vi "TestServerComm1.vi"() -> ()   [LabVIEW 2017]
uses:
  <vilib>/addons/InsightCM/MessageBus/Base/controls/ConnectionInfo.ctl
  <vilib>/NI/Software Watchdog/Pound/Pound.lvclass
  <vilib>/addons/Qbus/Qbus.lvclass
  <vilib>/addons/TraceLogger/TraceLogger.lvlib
  <vilib>/addons/InsightCM/Devices/Shared/Common/ServerComm/ServerComm.lvlib
  <vilib>/addons/TimerProcess/TimerProcess.lvlib
panel:
  out "log":i32(listbox)=-1
  in  "stop":bool
  in  "connection info":T1={"ClientName"="Bop9068", "TransceiverHost"="10.2.64.56", "TransceiverPort"=6342, "Password"="password"}
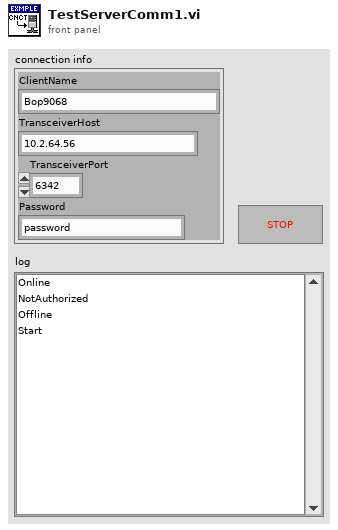
[diagram p1: front panel]
types:
  T1 = typedef "ConnectionInfo.ctl" = cluster{"ClientName":string, "TransceiverHost":string, "TransceiverPort":u16, "Password":string}
  T2 = typedef "ServerComm.lvlib/ConnectionStatus.ctl" = enum16{"Offline", "NotAuthorized", "Online"}
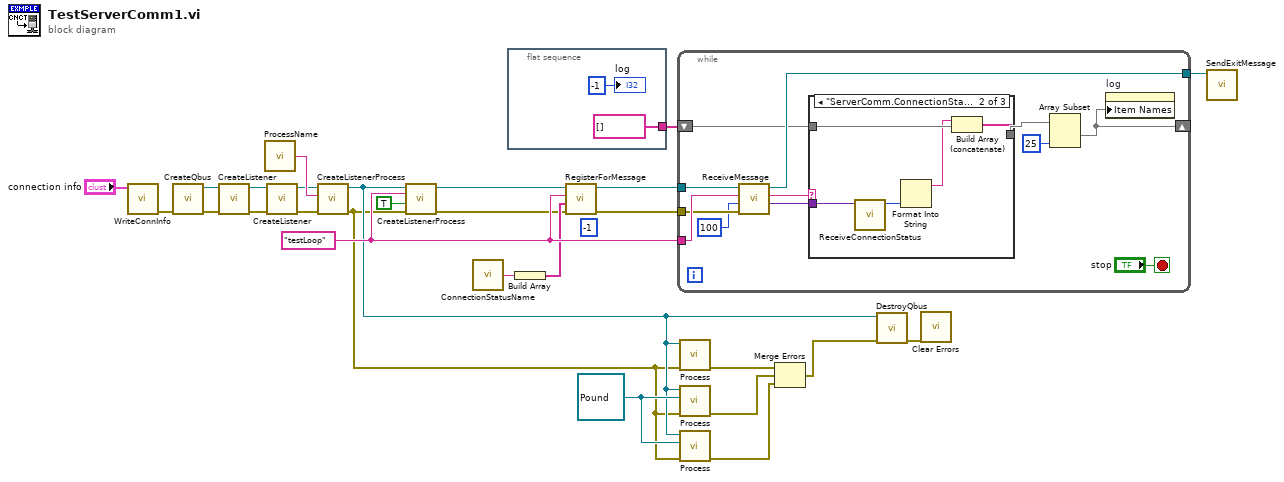
[diagram p0: block diagram]
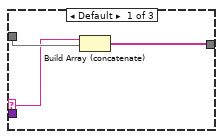
[diagram p2: hidden frame]
diagram:
  (unwired) -1 ("timeout (-1)")
  w14 = refnum<class "Pound.lvclass"> refnum ("Pound in")
  w17 = "testLoop" ("ProcessName")
  n1 = call <vilib>:"WriteConnInfo.vi"("connection info"="connection info") -> ("error out"=w22:errorcluster)  [unwired: 10 in]
  n2 = call <vilib>:"CreateQbus.vi"("error in (no error)"=w22) -> ("error out"=w11:errorcluster, "Qbus"=w12:refnum<class "Qbus.lvclass">)  [unwired: 9 in]
  n3 = call <vilib>:"CreateListener.vi"("error in (no error)"=w11, "Qbus in"=w12) -> ("error out"=w9:errorcluster, "Qbus out"=w10:refnum<class "Qbus.lvclass">)  [unwired: 8 in]
  n4 = call <vilib>:"ProcessName.vi"() -> ("process name"=w27:string)  [unwired: 5 in]
  n5 = call <vilib>:"CreateListener.vi"("error in (no error)"=w9, "qbus in"=w10) -> ("error out"=w7:errorcluster, "qbus out"=w8:refnum<class "Qbus.lvclass">)  [unwired: 8 in]
  n6 = call <vilib>:"CreateListenerProcess.vi"("error in (no error)"=w7, "process name"=w27, "Qbus in"=w8) -> ("error in (no error)"=w5:errorcluster, "Qbus out"=w6:refnum<class "Qbus.lvclass">)  [unwired: 7 in]
  n7 = call <vilib>:"CreateListenerProcess.vi"("error in (no error)"=w5, "master"=TRUE ("Master"), "process name"=w17, "Qbus in"=w6) -> ("error in (no error)"=w2:errorcluster, "Qbus out"=w1:refnum<class "Qbus.lvclass">)  [unwired: 6 in]
  n8 = call <vilib>:"ConnectionStatusName.vi"() -> ("message name"=w15:string)  [unwired: 5 in]
  n9 = flat-sequence {
    tunnel: [string[] []] -> w19
    frame #0 {
      "log" <- -1 ("Listbox")
    }
  }
  n10 = Build Array(w15) -> (w16:string[])
  n11 = call <vilib>:"RegisterForMessage.vi"("error in (no error)"=w2, "message names"=w16, "process name"=w17, "Qbus in"=w1) -> ("error in (no error)"=w3:errorcluster, "Qbus out"=w4:refnum<class "Qbus.lvclass">)  [unwired: 6 in]
  n12 = while {
    tunnel: w4 -> [w41]
    tunnel: w17 -> [w40]
    tunnel: w3 -> [w39]
    tunnel: [w35] -> w20
    shift-right: [w31] -> _
    shift-left: w19 -> [w34]
    stop <- "stop" stop-if-true
    n13 = call <vilib>:"ReceiveMessage.vi"("error in (no error)"=w39, "timeout (0)"=100, "process name"=w40, "Qbus in"=w41) -> ("message value"=w30:variant, "message name"=w36:string, "Qbus out"=w35:refnum<class "Qbus.lvclass">)  [unwired: 2 in, 3 out]
    n14 = case shown="\"ServerComm.ConnectionStatus\"" w36 {
      selector: w36 -> [w43 _ _]
      tunnel: [w42 w48 w50] -> w32
      tunnel: w34 -> [w44 w49 w50]
      tunnel: w30 -> [_ w46 _]
      frame Default {
        n15 = Build Array (concatenate)(w43, w44) -> (w42:string[])
      }
      frame "ServerComm.ConnectionStatus" {
        n16 = call <vilib>:"ReceiveConnectionStatus.vi"("body"=w46) -> ("status"=w45:T2)  [unwired: 7 in, 3 out]
        n17 = Format Into String(w45) -> (resulting string=w47:string)  [unwired: 3 in, 1 out]
        n18 = Build Array (concatenate)(w47, w49) -> (w48:string[])
      }
      frame "" {
      }
    }
    n19 = Array Subset(array=w32, length=25) -> (w31:string[])  [unwired: 1 in]
    n20 = property on="log" class="LstBox (strict)"("Item Names"=w31) -> ()  [unwired: 2 in, 2 out]
  }
  n21 = call <vilib>:"Process.vi"("error in (no error)"=w5, "qbus in"=w6) -> ("error out"=w25:errorcluster)  [unwired: 9 in]
  n22 = call <vilib>:"Process.vi"("error in (no error)"=w5, "Pound in"=w14, "Qbus in"=w6) -> ("error out"=w23:errorcluster)  [unwired: 8 in]
  n23 = call <vilib>:"Process.vi"("error in (no error)"=w5, "pound in"=w14, "qbus in"=w6) -> ("error out"=w13:errorcluster)  [unwired: 8 in]
  n24 = Merge Errors(w25, w23, w13) -> (w24:errorcluster)
  n25 = call <vilib>:"DestroyQbus.vi"("error in (no error)"=w24, "Qbus"=w6) -> ("error in (no error)"=w18:errorcluster)  [unwired: 9 in]
  n26 = call <vilib>:"Clear Errors.vi"("error in (no error)"=w18) -> ()  [unwired: 5 in, 2 out]
  n27 = call <vilib>:"SendExitMessage.vi"("Qbus in"=w20) -> ()  [unwired: 9 in, 2 out]
